vi "Convert chars to strings.vi"(10 "Char Array":i8[][](array[numeric]), 11 "Array Length":i32) -> (3 "Strings":string[](array[string]))   [LabVIEW 2023, in "Database.lvlib"]
uses:
  Database.lvlib
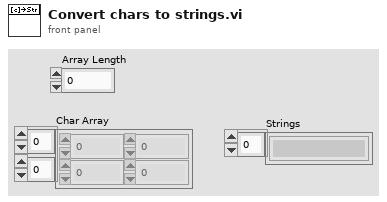
[diagram p1: front panel]
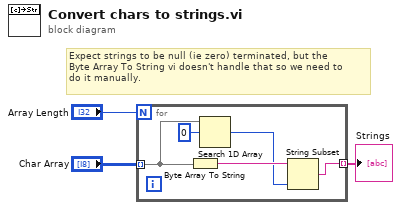
[diagram p0: block diagram]
diagram:
  # "Expect strings to be null (ie zero) terminated, but the\nByte Array To String vi doesn't handle that so we need to \ndo it manually."
  n1 = for {
    N: "Array Length" -> [_]
    tunnel: "Char Array" -> [w8] mode=indexing
    tunnel: [w5] -> w1 mode=indexing
    n2 = Byte Array To String(unsigned byte array=w8) -> (string=w6:string)
    n3 = Search 1D Array(1D array=w8, element=i8 0) -> (index of element=w4:i32)  [unwired: 1 in]
    n4 = String Subset(string=w6, length (rest)=w4) -> (substring=w5:string)  [unwired: 1 in]
  }
  "Strings" <- w1
